vi "CANFD Get Diagnostic.vi"(8 "error in (no error)":errorcluster, 9 "pCanDiagnostic":T1, 10 "CANIndex":u8, 11 "DevHandle":i32) -> (0 "error out":errorcluster, 1 "pCanDiagnostic out":T1, 3 "function return":i32)   [LabVIEW 2010, in "usb2canfd.lvlib"]
doc: "int WINAPI CANFD_GetDiagnostic(int DevHandle, unsigned char CANIndex, CANFD_DIAGNOSTIC *pCanDiagnostic);"
uses:
  usb2canfd.lvlib
  USB2XXX/trunk/USB2XXX/USB2XXX/vs2010/Release/USB2XXX.dll
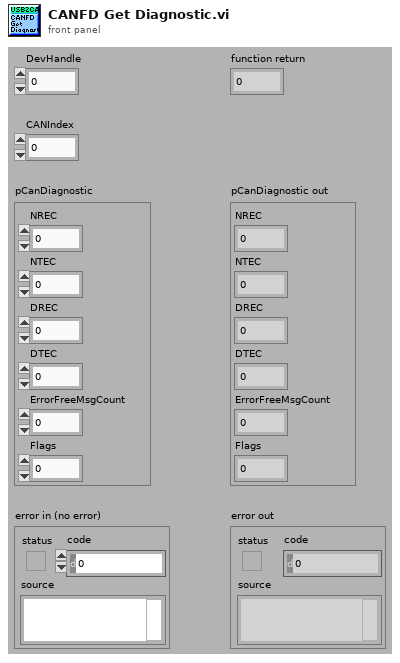
[diagram p1: front panel]
types:
  T1 = cluster{"NREC":u8, "NTEC":u8, "DREC":u8, "DTEC":u8, "ErrorFreeMsgCount":u16, "Flags":u16}
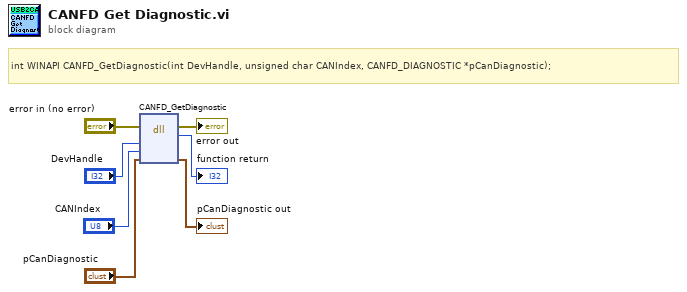
[diagram p0: block diagram]
diagram:
  # "int WINAPI CANFD_GetDiagnostic(int DevHandle, unsigned char CANIndex, CANFD_DIAGNOSTIC *pCanDiagnostic);"
  n1 = dll-call lib="E:/OtherWork/STM32/USB2XXX/trunk/USB2XXX/USB2XXX/vs2010/Release/USB2XXX.*" fn="CANFD_GetDiagnostic"(error in="error in (no error)", "DevHandle"="DevHandle", "CANIndex"="CANIndex", "pCanDiagnostic"="pCanDiagnostic") -> (error out=→"error out":errorcluster, →"function return":i32, "pCanDiagnostic"=→"pCanDiagnostic out":T1)  [unwired: 4 in, 1 out]
